vi "StartupVI_Globals.vi"() -> ()   [LabVIEW 2015]
panel:
  in  "Startup VIs":path[](array[path])=[path "C:/Users/Public/Documents/National Instruments/AndorAcquire/NIDAQControls/NIDAQControl2.vi", path "C:/Users/Public/Documents/National Instruments/AndorAcquire/Andor/LiveAcquire.vi", path "C:/Users/Public/Documents/National Instruments/AndorAcquire/Andor/WriteData.vi"]
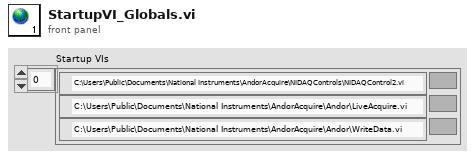
[diagram p1: front panel]
diagram:
